vi "GEA3 Read Mix Valve Position.vi"(8 "error in (no error)":errorcluster, 10 "GEA Inputs":T1 {"Destination" format="%.0x"; "Source" format="%.0x"}, 11 ".NET Refnum in":refnum<k24>) -> (0 "error out":errorcluster, 2 "Mix Valve Position":i16, 3 ".NET Refnum out":refnum<k24>)   [LabVIEW 2016]
uses:
  C:/TechnologyLab/NI-2010/Drivers/GEA3 Toolkit/GEA3 DLL Source/GeaCommunication.dll
  GEA3 DLL Source/GeaCommunication.dll
  type defs/Source_Destination.ctl
  type defs/ERD Read Data In.ctl
  type defs/Data Type.ctl
  library/GEA2_Toolkit.lvlib
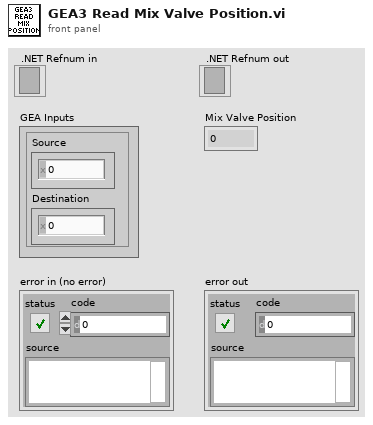
[diagram p1: front panel]
types:
  T1 = typedef "GEA2_Toolkit.lvlib/Source_Destination.ctl" = cluster{"Source":u8, "Destination":u8}
  T2 = typedef "GEA2_Toolkit.lvlib/ERD Read Data In.ctl" = cluster{"ERD Number":u16, "Data Type":T3}
  T3 = typedef "GEA2_Toolkit.lvlib/Data Type.ctl" = enum16{"string", "boolean", "uint8_t", "uint16_t", "uint32_t", "uint64_t", "int8_t", "int16_t", "int32_t", "int64_t"}
  T4 = typedef "GEA2_Toolkit.lvlib/ERD Read Data Out.ctl" = cluster{"ERD Number":u16, "Data":string}
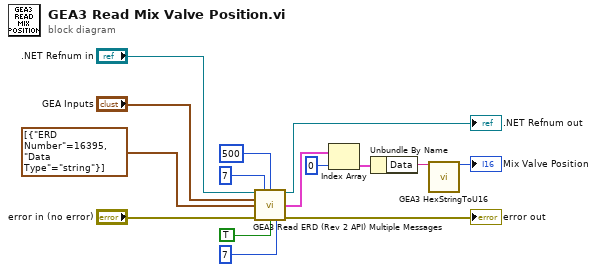
[diagram p0: block diagram]
diagram:
  n1 = call "GEA3 Read ERD (Rev 2 API) Multiple Messages.vi"("GEA2 Reference In"=".NET Refnum in", "Retry Count"=7, "Read Timeout (ms)"=u32 500, "GEA Inputs"="GEA Inputs", "Read ERD List"=T2[] [{"ERD Number"=16395, "Data Type"=enum."string"}], "Error In"="error in (no error)", "Verify ERD Response?"=TRUE, "Low Level Retry Count"=u8 7) -> ("GEA2 Reference Out"=→".NET Refnum out":refnum<k24>, "ERD Data Out"=w10:T4[], "Error Out"=→"error out":errorcluster)  [unwired: 4 in, 1 out]
  n2 = Index Array(array=w10, index=0) -> (element=w12:T4)
  n3 = Unbundle By Name(w12) -> ("Data"=w13:string)
  n4 = call "GEA3 HexStringToU16.vi"("Input String"=w13) -> ("Number Out"=→"Mix Valve Position":u16)  [unwired: 14 in]
